vi "pH电极校准.vi"() -> ()   [LabVIEW 2016, in "斯坦道多参数.lvlib"]
uses:
  <vilib>/Utility/miscctls.llb/LVPointTypeDef.ctl
  <vilib>/Analysis/NI_AALBase.lvlib
panel:
  in  "刷新按钮":bool
  out "第三点信号值":dbl
  out "第二点信号值":dbl
  out "第一点信号值":dbl
  out "温度":dbl format="%#.2f"
  out "通讯状态":string
  out "电极状态标志":u16(ring) items=["OK", "第一点校正通过", "第二点校正通过", "校正失败,电极零点超出范围", "校正失败,电极斜率超出范围", "第三点校正通过"]
  in  "三点标液3":u16(ring)=6 caption="标液3" items=["TECH4.00", "TECH7.00", "TECH10.00", "NIST1.68", "NIST4.01", "NIST6.86", "NIST9.18", "NIST12.68"]
  in  "三点标液2":u16(ring)=5 caption="标液2" items=["TECH4.00", "TECH7.00", "TECH10.00", "NIST1.68", "NIST4.01", "NIST6.86", "NIST9.18", "NIST12.68"]
  in  "三点标液1":u16(ring)=4 caption="标液1" items=["TECH4.00", "TECH7.00", "TECH10.00", "NIST1.68", "NIST4.01", "NIST6.86", "NIST9.18", "NIST12.68"]
  out "第三点校准值":dbl
  in  "校准停止":bool
  in  "校准启动":bool
  out "第二点校准值":dbl
  out "第一点校准值":dbl
  out "提示":string
  in  "校准模式":enum16{"两点校准", "单点校准", "三点校准"}(ring)
  out "最小值":sgl format="%#.2f"
  out "最大值":sgl format="%#.2f"
  out "变异系数":dbl format="%#.6f"
  out "standard deviation":dbl caption="标准差" format="%#.2f"
  out "mean":dbl caption="均值" format="%#.2f"
  out "波形图表":sgl(graph) caption="历史曲线"
  out "当前检测值":dbl caption="测量值" format="%#.2f"
  out "标液2":dbl
  out "标液1":dbl
  out "当前信号值":dbl caption="信号值" format="%#.2f"
  out "偏移值补偿":dbl caption="pH偏移修正值" format="%#.2f"
  out "电极斜率":dbl format="%#.6f"
  out "电极零点":dbl format="%#.6f"
  # "酸碱度电极设定"
  # "℃"
  # "mV"
  # "mV"
  # "%"
  # "请选择校准模式:"
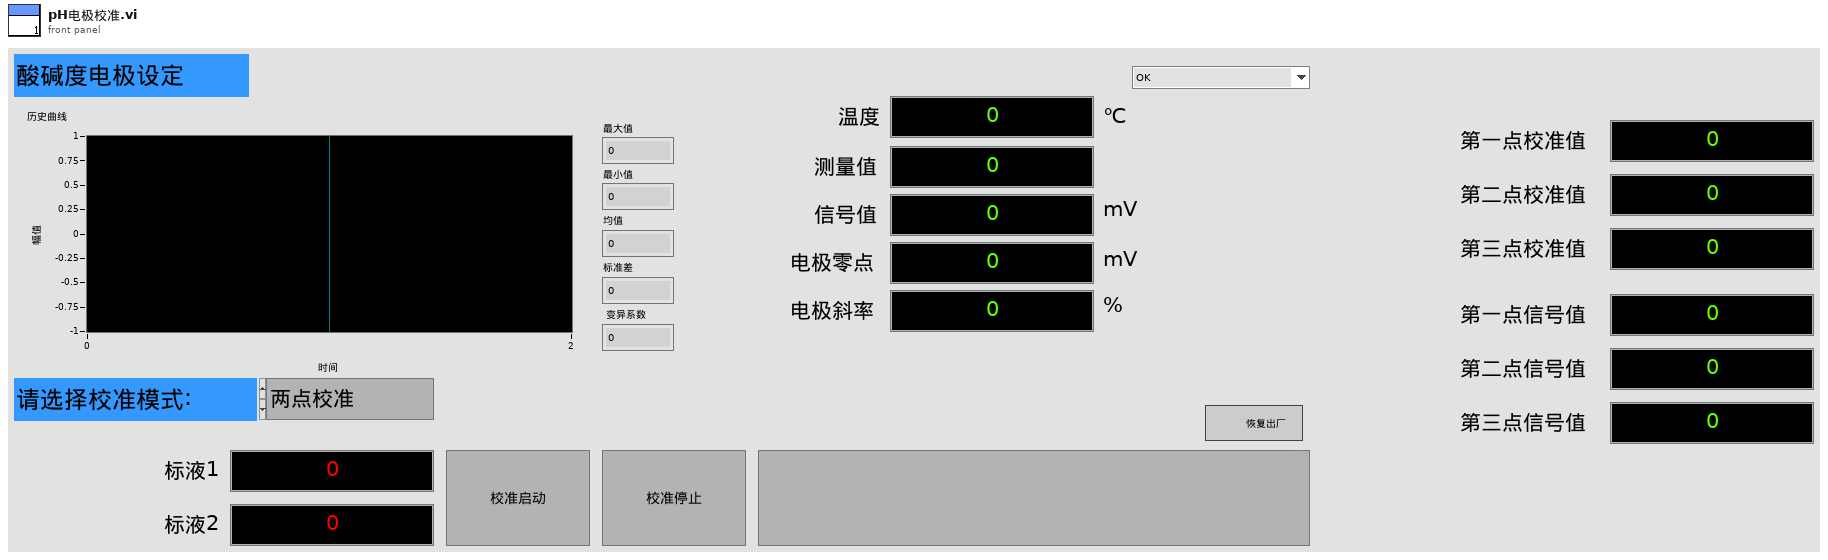
[diagram p1: front panel]
types:
  T1 = typedef "LVPointTypeDef.ctl" = cluster{"Horizontal":i16, "Vertical":i16}
  T2 = enum8{"Enabled", "Disabled", "Disabled and Grayed Out"}
  T3 = cluster{"电极状态标志":u16, "电极型号标志":u16, "酸碱度测量值":sgl, "温度测量值":sgl, "酸碱度信号值":sgl, "温度信号值":sgl, "酸碱度偏移修正值":sgl, "温度偏移修正值":sgl, "手动温度补偿值":sgl, "酸碱度电极零点":sgl, "酸碱度电极斜率":sgl, "第1点标准值记录":sgl, "第1点信号值记录":sgl, "第1点温度值记录":sgl, "第2点标准值记录":sgl, "第2点信号值记录":sgl, "第2点温度值记录":sgl, "命令滤波设定":u16, "温度模式":enum16{"ATC", "MTC"}, "生产批次":u16, "电极序号":u16, "串口地址":u16, "串口波特率":enum16{"9600", "19200", "115200"}, "串口校验位":enum16{"NONE", "ODD", "EVEN"}, "串口停止位":enum16{"1bit", "2bit"}, "第一点标准值":sgl, "第二点标准值":sgl}
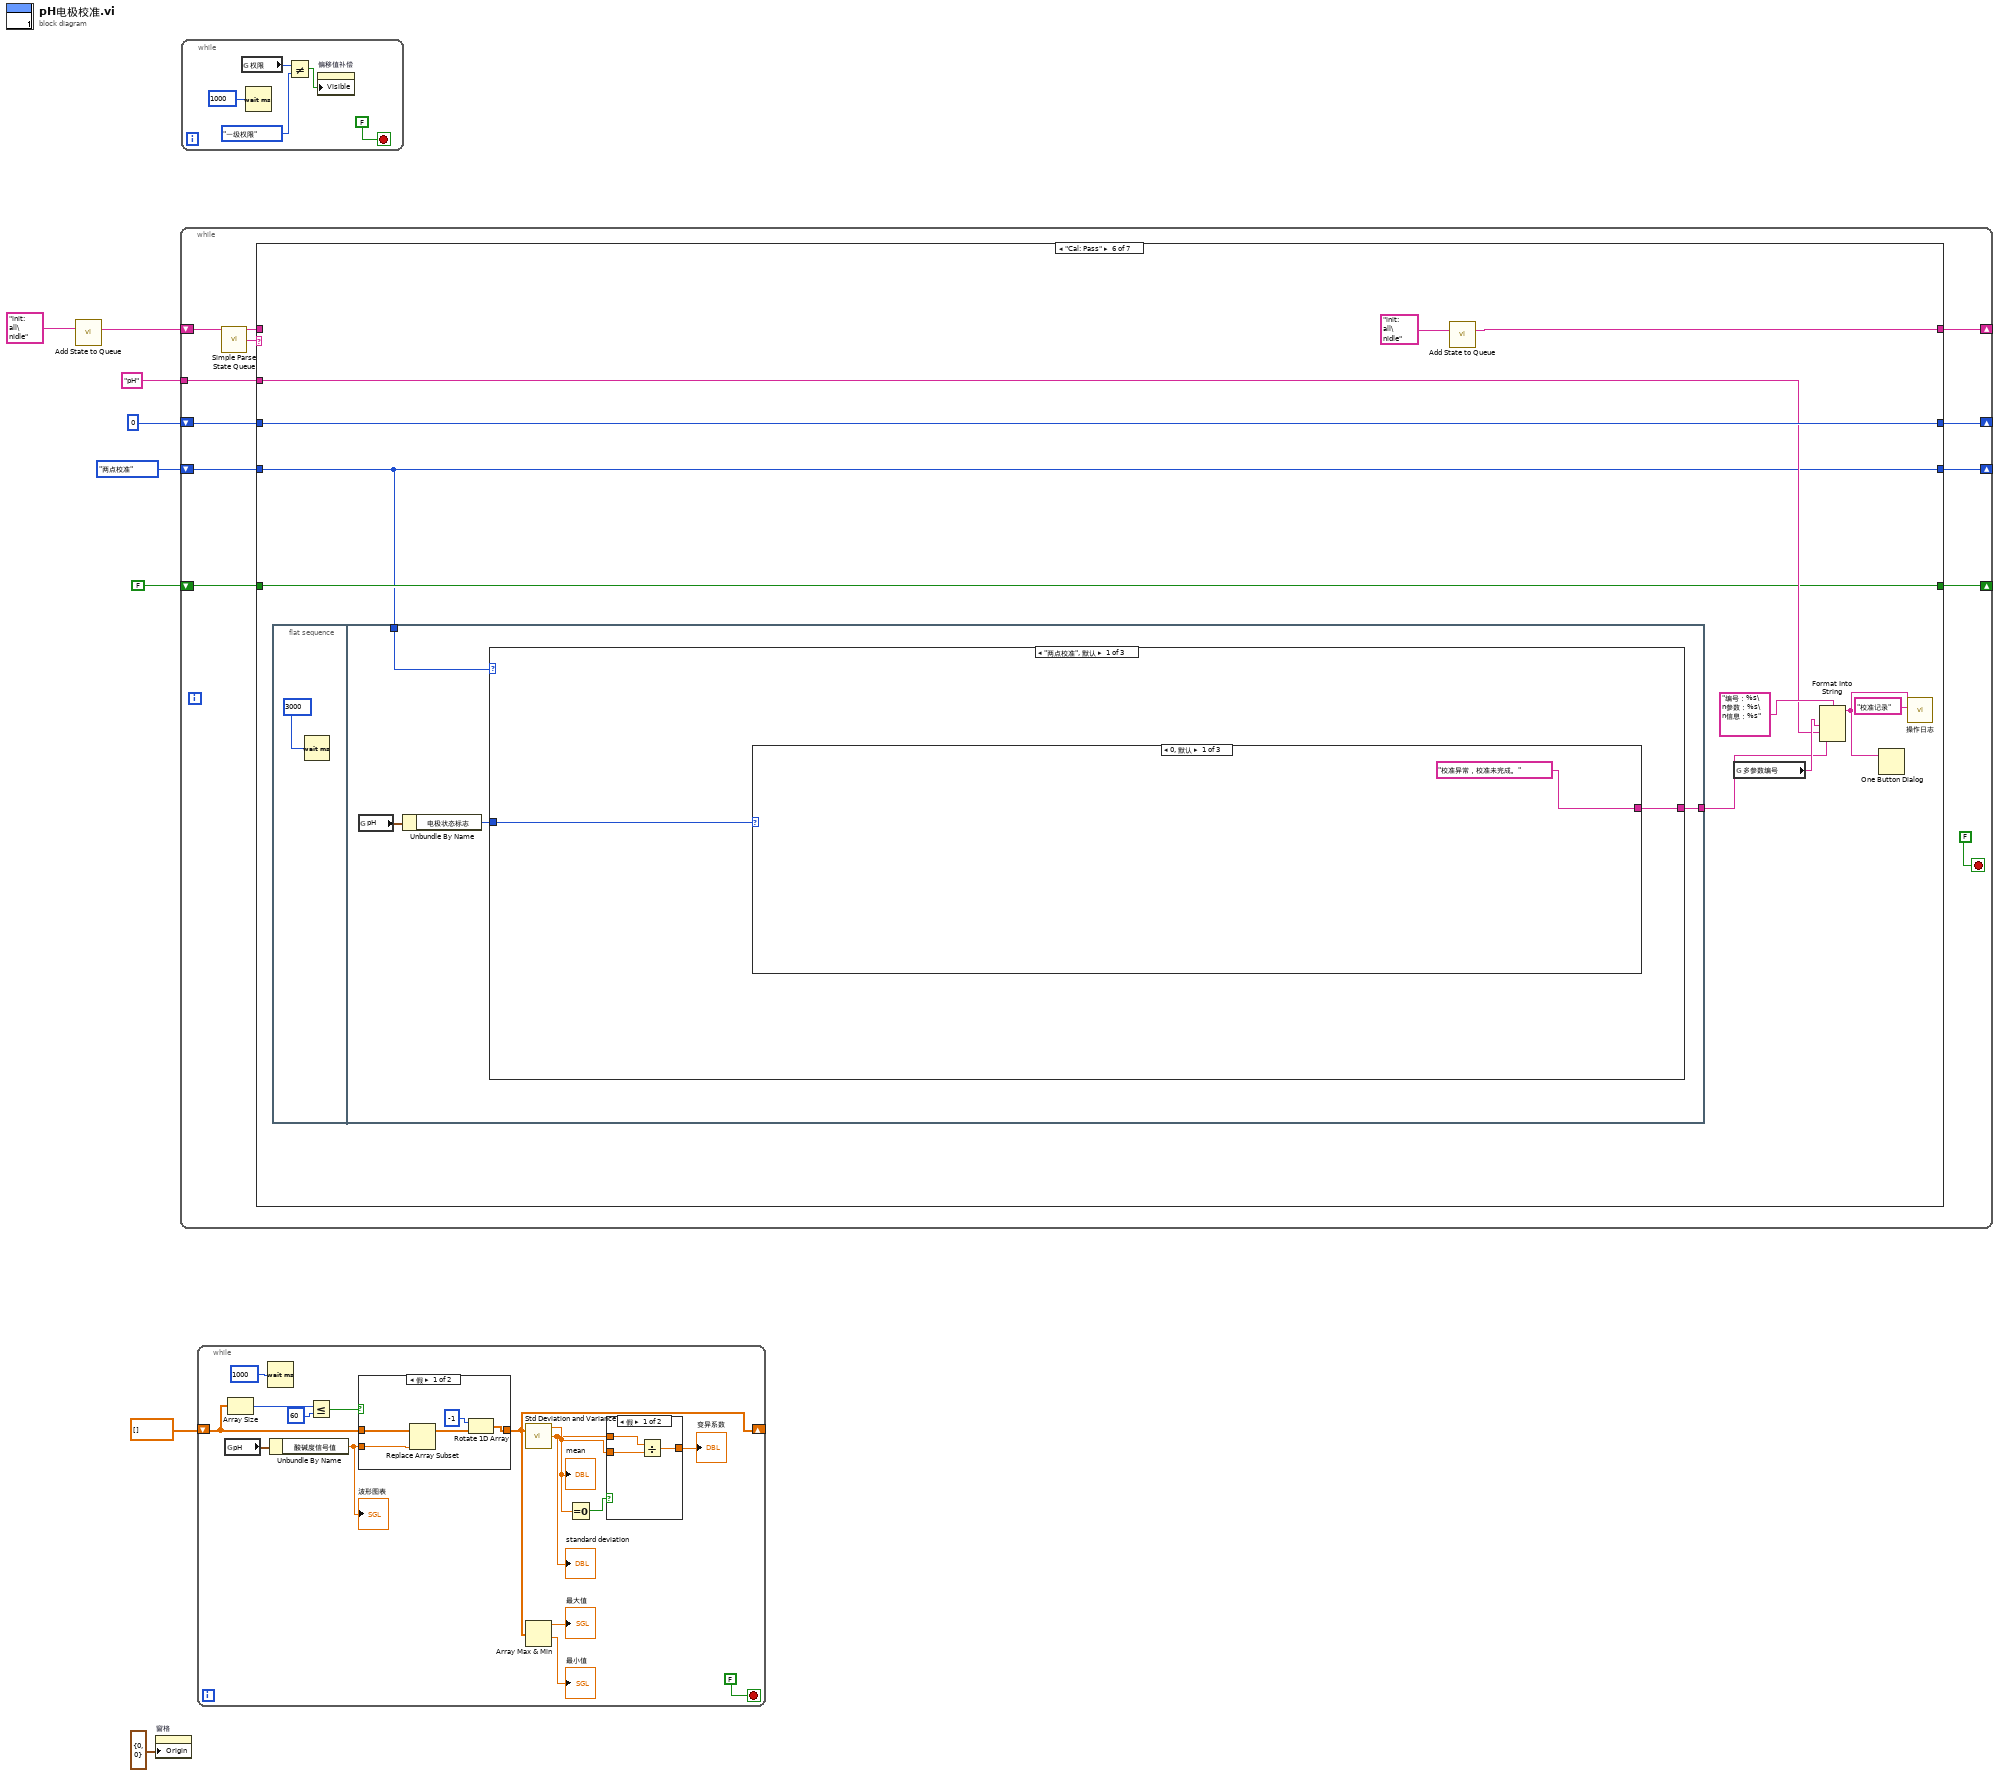
[diagram p0: block diagram]
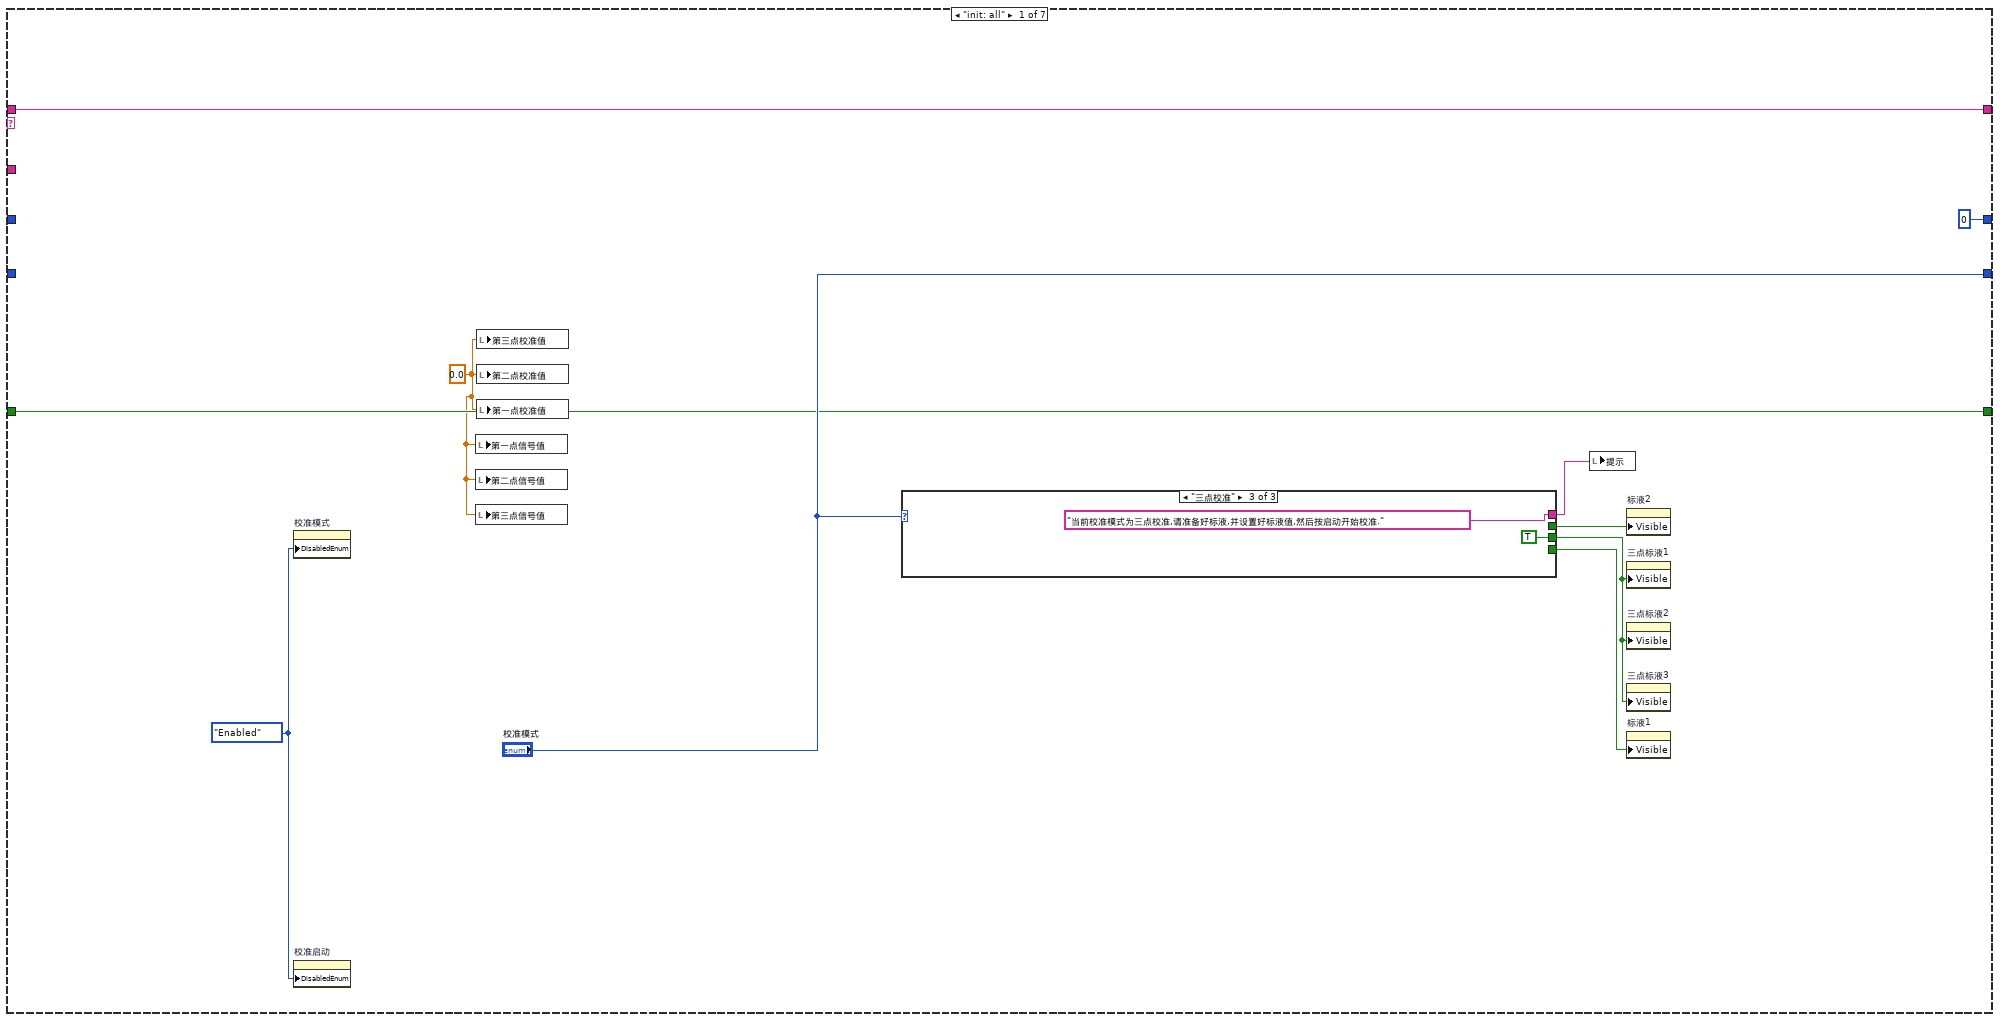
[diagram p2: hidden frame]
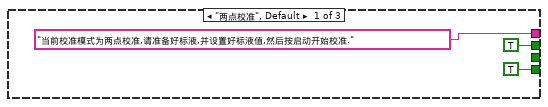
[diagram p3: hidden frame]
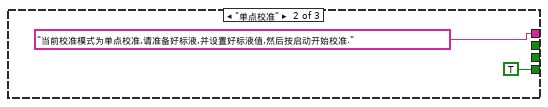
[diagram p4: hidden frame]
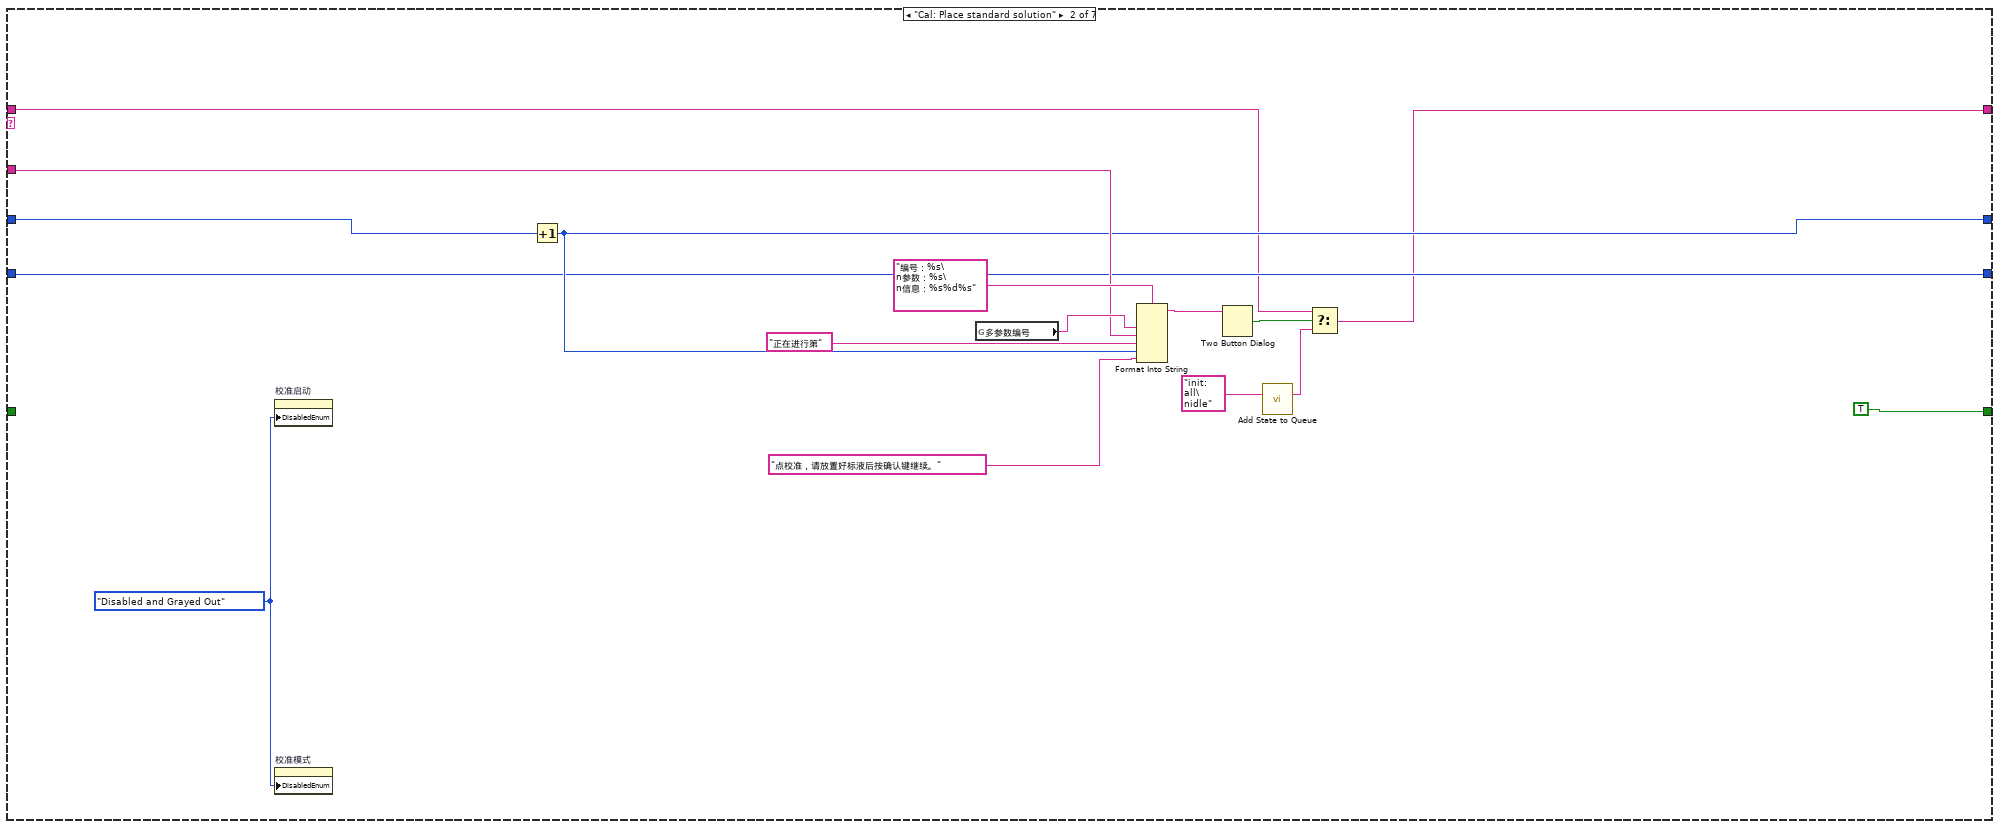
[diagram p5: hidden frame]
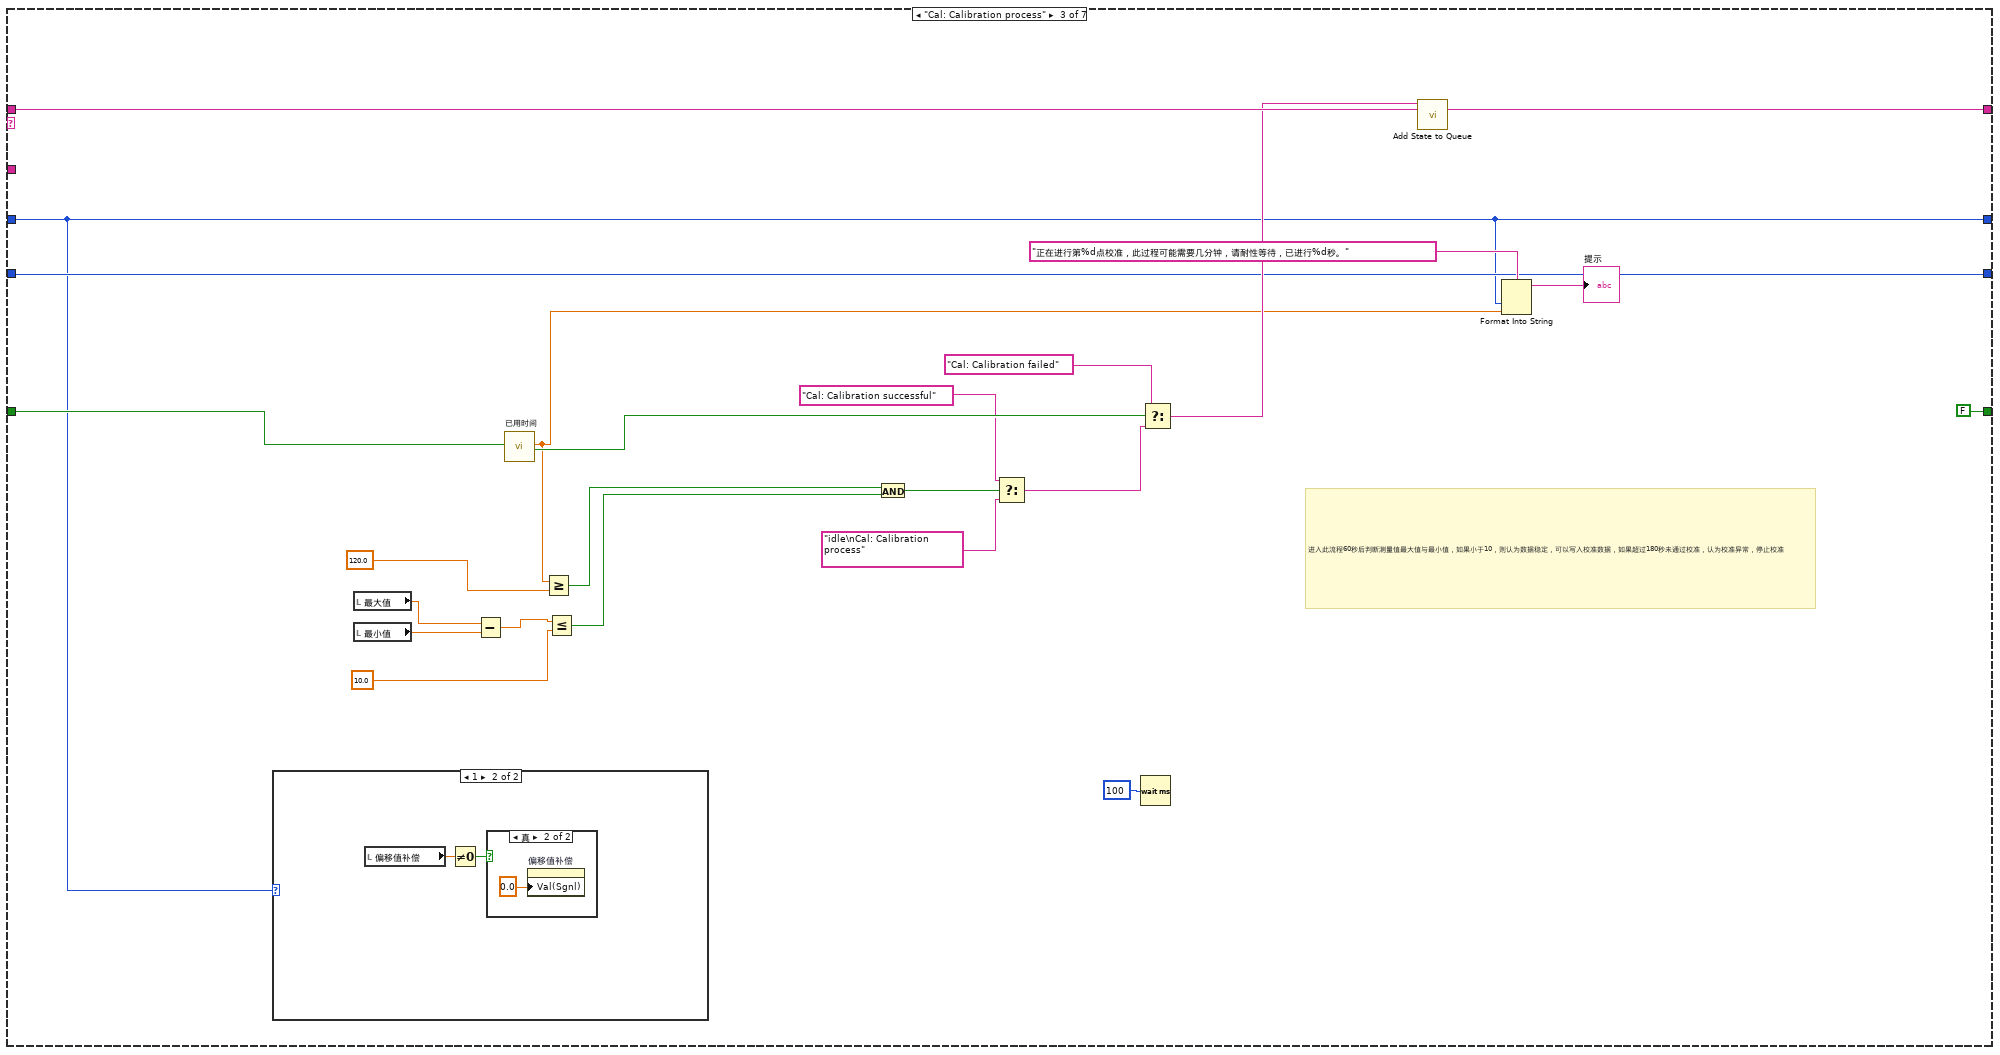
[diagram p6: hidden frame]
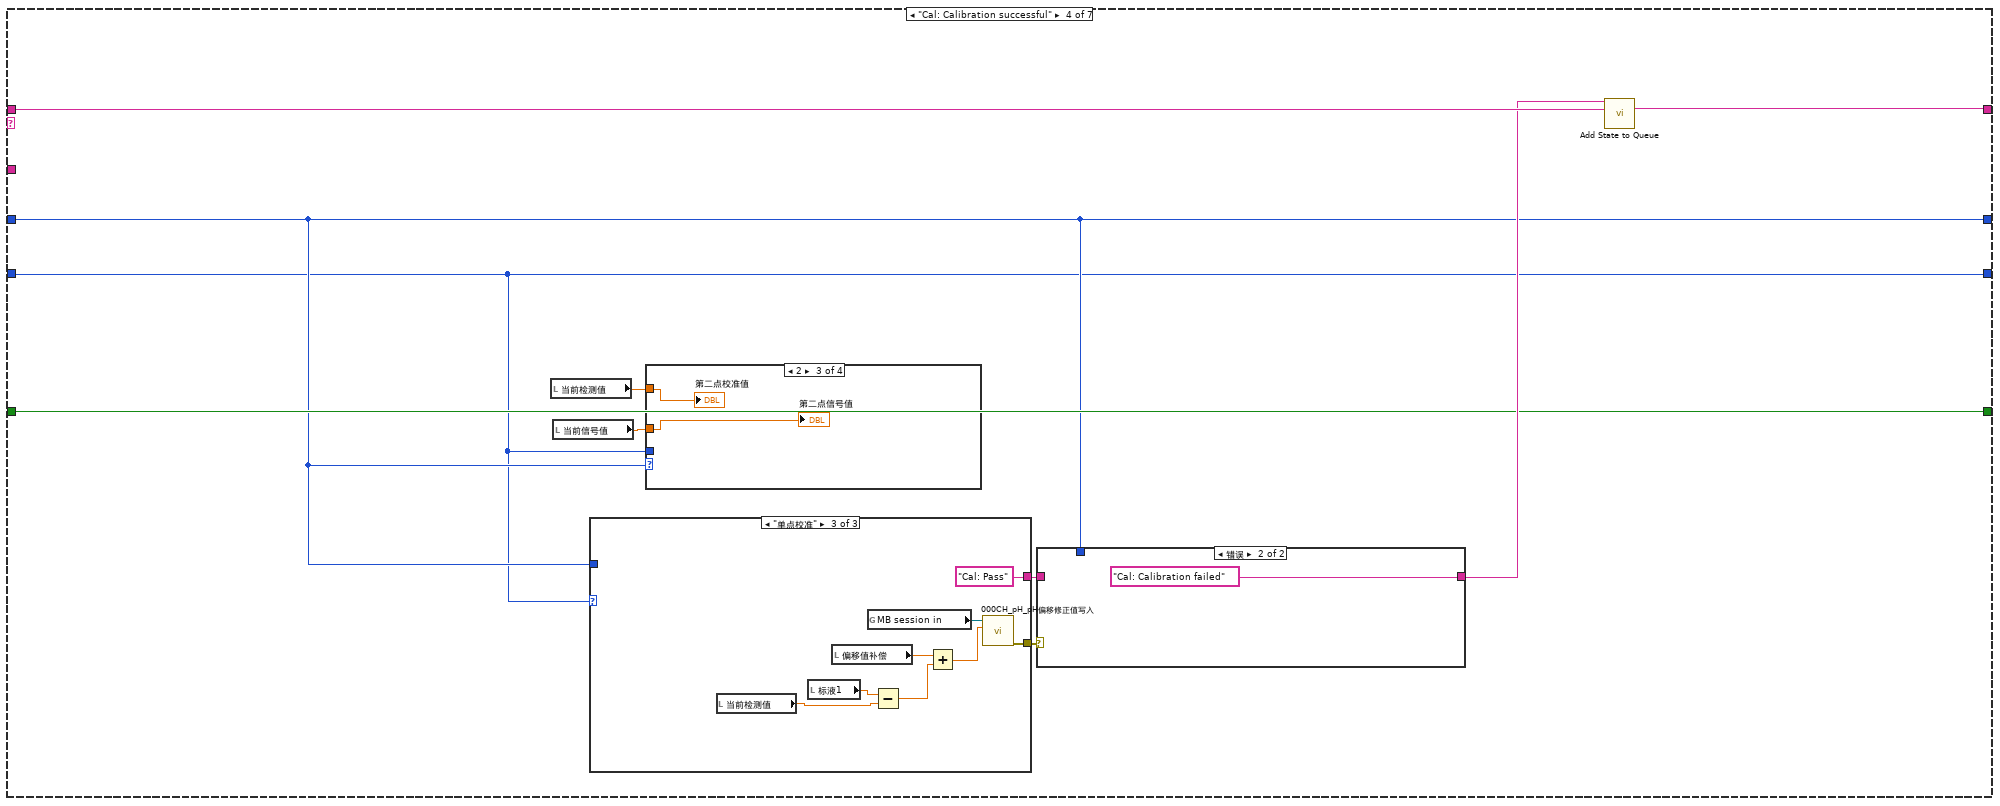
[diagram p9: hidden frame]
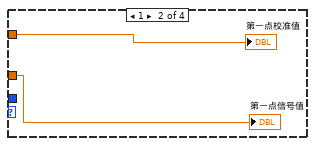
[diagram p11: hidden frame]
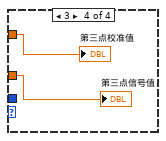
[diagram p12: hidden frame]
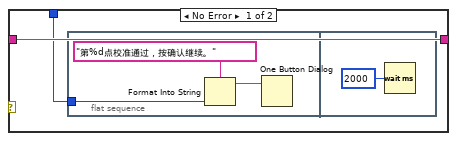
[diagram p13: hidden frame]
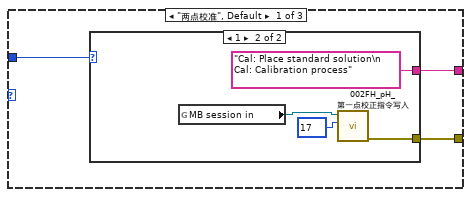
[diagram p14: hidden frame]
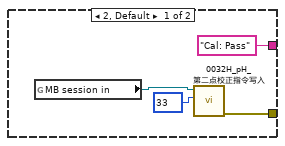
[diagram p15: hidden frame]
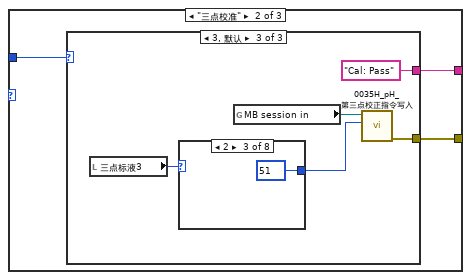
[diagram p16: hidden frame]
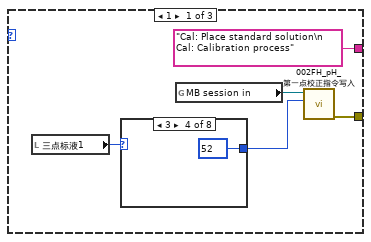
[diagram p17: hidden frame]
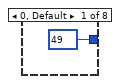
[diagram p18: hidden frame]
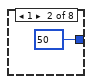
[diagram p19: hidden frame]
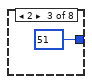
[diagram p20: hidden frame]
diagram:
  n1 = call "Add State to Queue.vi"("State(s) In (\"\")"="init: all\nidle" ("State(s) In (\"\")")) -> ("States Out"=w5:string)  [unwired: 14 in]
  n2 = property on="窗格" class="Pane"("Origin"=T1 {"Horizontal"=0, "Vertical"=0} ("原点")) -> ()  [unwired: 2 in, 2 out]
  n3 = while {
    shift-right: [w16] -> _
    shift-left: w5 -> [w20]
    shift-right: [w13] -> _
    shift-left: 0 -> [w15]
    tunnel: "pH" ("State(s) In (\"\")") -> [w14]
    shift-right: [w11] -> _
    shift-left: enum16{"两点校准", "单点校准", "三点校准"}."两点校准" ("校准模式") -> [w12]
    shift-right: [w9] -> _
    shift-left: FALSE -> [w10]
    stop <- FALSE stop-if-true
    n4 = call "Simple Parse State Queue.vi"("State Queue"=w20) -> ("Remain States"=w17:string, "Next State"=w18:string)  [unwired: 13 in]
    n5 = case shown="\"Cal: Pass\"" w18 {
      tunnel: w17 -> [w30 w39 w72 w88 _ _ w232]
      tunnel: [w30 w38 w71 w87 w172 w176 w231] -> w16
      tunnel: w15 -> [_ w49 w55 w82 w175 w186 w229]
      tunnel: w14 -> [_ w50 _ _ w165 w182 _]
      tunnel: [0 w47 w55 w82 w175 w186 w230] -> w13
      tunnel: w12 -> [_ w46 w56 w81 w174 w178 w228]
      tunnel: ["校准模式" w46 w56 w81 w174 w178 w228] -> w11
      tunnel: w10 -> [w23 _ w58 w83 w173 w181 w226]
      tunnel: [w23 TRUE FALSE w83 w173 w181 w226] -> w9
      frame "init: all" {
        w22 = T2."Enabled" ("禁用")
        w21 = 0.0 ("第一点校准值")
        n6 = property on="校准模式" class="Enum (严格)"("DisabledEnum"=w22) -> ()  [unwired: 2 in, 2 out]
        n7 = property on="校准启动" class="Bool"("DisabledEnum"=w22) -> ()  [unwired: 2 in, 2 out]
        n8 = local write "第一点信号值"(w21) -> ()
        n9 = local write "第二点信号值"(w21) -> ()
        n10 = local write "第三点信号值"(w21) -> ()
        n11 = local write "第三点校准值"(w21) -> ()
        n12 = local write "第二点校准值"(w21) -> ()
        n13 = local write "第一点校准值"(w21) -> ()
        n14 = case shown="\"三点校准\"" "校准模式" {
          tunnel: ["当前校准模式为两点校准,请准备好标液,并设置好标液值,然后按启动开始校准." ("提示") "当前校准模式为单点校准,请准备好标液,并设置好标液值,然后按启动开始校准." ("提示") "当前校准模式为三点校准,请准备好标液,并设置好标液值,然后按启动开始校准." ("提示")] -> w25
          tunnel: [TRUE ("可见") _ _] -> w29
          tunnel: [TRUE ("可见") TRUE ("可见") _] -> w27
          tunnel: [_ _ TRUE ("可见")] -> w28
          frame "两点校准", Default {
          }
          frame "单点校准" {
          }
          frame "三点校准" {
          }
        }
        n15 = local write "提示"(w25) -> ()
        n16 = property on="标液2" class="DigNum (严格)"("Visible"=w29) -> ()  [unwired: 2 in, 2 out]
        n17 = property on="三点标液1" class="Ring (严格)"("Visible"=w28) -> ()  [unwired: 2 in, 2 out]
        n18 = property on="三点标液2" class="Ring (严格)"("Visible"=w28) -> ()  [unwired: 2 in, 2 out]
        n19 = property on="三点标液3" class="Ring (严格)"("Visible"=w28) -> ()  [unwired: 2 in, 2 out]
        n20 = property on="标液1" class="DigNum (严格)"("Visible"=w27) -> ()  [unwired: 2 in, 2 out]
      }
      frame "Cal: Place standard solution" {
        w44 = T2."Disabled and Grayed Out" ("禁用")
        n21 = property on="校准启动" class="Bool"("DisabledEnum"=w44) -> ()  [unwired: 2 in, 2 out]
        n22 = property on="校准模式" class="Enum (严格)"("DisabledEnum"=w44) -> ()  [unwired: 2 in, 2 out]
        n23 = Increment(x=w49) -> (x+1=w47:i32)
        n24 = global read "多参数全局变量.vi" "多参数编号"() -> (w52:string)
        n25 = Format Into String(format string="编号：%s\n参数：%s\n信息：%s%d%s" ("格式字符串"), w52, w50, "正在进行第" ("消息"), w47, "点校准，请放置好标液后按确认键继续。" ("消息")) -> (resulting string=w43:string)  [unwired: 2 in, 1 out]
        n26 = Two Button Dialog(message=w43) -> (T button?=w42:bool)  [unwired: 2 in]
        n27 = call "Add State to Queue.vi"("State(s) In (\"\")"="init: all\nidle" ("State(s) In (\"\")")) -> ("States Out"=w40:string)  [unwired: 14 in]
        n28 = Select(t=w39, s=w42, f=w40) -> (s? t:f=w38:string)
      }
      frame "Cal: Calibration process" {
        # "进入此流程60秒后判断测量值最大值与最小值，如果小于10，则认为数据稳定，可以写入校准数据，如果超过180秒未通过校准，认为校准异常，停止校准"
        n29 = case shown="1" w55 {
          frame 0, Default {
          }
          frame 1 {
            n30 = local read "偏移值补偿"() -> (w78:dbl)
            n31 = Not Equal To 0?(x=w78) -> (x != 0?=w79:bool)
            n32 = case shown="真" w79 {
              frame False {
              }
              frame True {
                n33 = property on="偏移值补偿" class="DigNum (严格)"("Val(Sgnl)"=0.0 ("值(信号)")) -> ()  [unwired: 2 in, 2 out]
              }
            }
          }
        }
        n34 = local read "最大值"() -> (w76:sgl)
        n35 = local read "最小值"() -> (w75:sgl)
        n36 = Subtract(x=w76, y=w75) -> (x-y=w77:sgl)
        n37 = call "已用时间"("Reset"=w58) -> ("Elapsed Time (s)"=w54:dbl, "Time has Elapsed"=w73:bool)  [unwired: 11 in, 6 out]
        n38 = Greater Or Equal?(x=w54, y=120.0) -> (x >= y?=w68:bool)
        n39 = Less Or Equal?(x=w77, y=10.0) -> (x <= y?=w64:bool)
        n40 = And(x=w68, y=w64) -> (x .and. y?=w65:bool)
        n41 = Select(t="Cal: Calibration successful" ("State(s) In (\"\")"), s=w65, f="idle\nCal: Calibration process" ("State(s) In (\"\")")) -> (s? t:f=w63:string)
        n42 = Wait (ms)(milliseconds to wait=u32 100 ("等待时间（毫秒）")) -> ()  [unwired: 1 out]
        n43 = Select(t="Cal: Calibration failed" ("State(s) In (\"\")"), s=w73, f=w63) -> (s? t:f=w62:string)
        n44 = call "Add State to Queue.vi"("State(s) In Front (\"\")"=w62, "State(s) In (\"\")"=w72) -> ("States Out"=w71:string)  [unwired: 13 in]
        n45 = Format Into String(format string="正在进行第%d点校准，此过程可能需要几分钟，请耐性等待，已进行%d秒。" ("格式字符串"), w55, w54) -> (resulting string=→"提示":string)  [unwired: 2 in, 1 out]
      }
      frame "Cal: Calibration successful" {
        n46 = local read "当前检测值"() -> (w84:dbl)
        n47 = local read "当前信号值"() -> (w85:dbl)
        n48 = case shown="\"单点校准\"" w81 {
          tunnel: [w106 w117 w159] -> w90
          tunnel: [w105 w115 "Cal: Pass" ("State(s) In (\"\")")] -> w89
          tunnel: w82 -> [w104 w116 _]
          frame "两点校准", Default {
            n49 = case shown="1" w104 {
              tunnel: [w107 w112] -> w106
              tunnel: ["Cal: Pass" ("State(s) In (\"\")") "Cal: Place standard solution\n Cal: Calibration process" ("State(s) In (\"\")")] -> w105
              frame 2, Default {
                n50 = global read "多参数全局变量.vi" "MB session in"() -> (w109:refnum<class "MB_Master.lvclass">)
                n51 = call "0032H_pH_第二点校正指令写入.vi"("数值"=u16 33, "MB session in"=w109) -> ("error out"=w107:errorcluster)  [unwired: 8 in, 1 out]
              }
              frame 1 {
                n52 = global read "多参数全局变量.vi" "MB session in"() -> (w114:refnum<class "MB_Master.lvclass">)
                n53 = call "002FH_pH_第一点校正指令写入.vi"("数值"=u16 17, "MB session in"=w114) -> ("error out"=w112:errorcluster)  [unwired: 8 in, 1 out]
              }
            }
          }
          frame "三点校准" {
            n54 = case shown="3, 默认" w116 {
              tunnel: [w119 w132 w145] -> w117
              tunnel: ["Cal: Place standard solution\n Cal: Calibration process" ("State(s) In (\"\")") "Cal: Place standard solution\n Cal: Calibration process" ("State(s) In (\"\")") "Cal: Pass" ("State(s) In (\"\")")] -> w115
              frame 1 {
                n55 = local read "三点标液1"() -> (w121:u16)
                n56 = case shown="3" w121 {
                  tunnel: [u16 49 ("数值") u16 50 ("数值") u16 51 ("数值") u16 52 ("数值") u16 53 ("数值") u16 54 ("数值") u16 55 ("数值") u16 56 ("数值")] -> w120
                  frame 0, Default {
                  }
                  frame 1 {
                  }
                  frame 2 {
                  }
                  frame 3 {
                  }
                  frame 4 {
                  }
                  frame 5 {
                  }
                  frame 6 {
                  }
                  frame 7 {
                  }
                }
                n57 = global read "多参数全局变量.vi" "MB session in"() -> (w122:refnum<class "MB_Master.lvclass">)
                n58 = call "002FH_pH_第一点校正指令写入.vi"("数值"=w120, "MB session in"=w122) -> ("error out"=w119:errorcluster)  [unwired: 8 in, 1 out]
              }
              frame 2 {
                n59 = local read "三点标液2"() -> (w134:u16)
                n60 = case shown="7" w134 {
                  tunnel: [u16 49 ("数值") u16 50 ("数值") u16 51 ("数值") u16 52 ("数值") u16 53 ("数值") u16 54 ("数值") u16 55 ("数值") u16 56 ("数值")] -> w133
                  frame 0, Default {
                  }
                  frame 1 {
                  }
                  frame 2 {
                  }
                  frame 3 {
                  }
                  frame 4 {
                  }
                  frame 5 {
                  }
                  frame 6 {
                  }
                  frame 7 {
                  }
                }
                n61 = global read "多参数全局变量.vi" "MB session in"() -> (w135:refnum<class "MB_Master.lvclass">)
                n62 = call "0032H_pH_第二点校正指令写入.vi"("数值"=w133, "MB session in"=w135) -> ("error out"=w132:errorcluster)  [unwired: 8 in, 1 out]
              }
              frame 3, Default {
                n63 = local read "三点标液3"() -> (w147:u16)
                n64 = case shown="2" w147 {
                  tunnel: [u16 49 ("数值") u16 50 ("数值") u16 51 ("数值") u16 52 ("数值") u16 53 ("数值") u16 54 ("数值") u16 55 ("数值") u16 56 ("数值")] -> w146
                  frame 0, Default {
                  }
                  frame 1 {
                  }
                  frame 2 {
                  }
                  frame 3 {
                  }
                  frame 4 {
                  }
                  frame 5 {
                  }
                  frame 6 {
                  }
                  frame 7 {
                  }
                }
                n65 = global read "多参数全局变量.vi" "MB session in"() -> (w148:refnum<class "MB_Master.lvclass">)
                n66 = call "0035H_pH_第三点校正指令写入.vi"("数值"=w146, "MB session in"=w148) -> ("error out"=w145:errorcluster)  [unwired: 8 in, 1 out]
              }
            }
          }
          frame "单点校准" {
            n67 = local read "当前检测值"() -> (w157:dbl)
            n68 = local read "标液1"() -> (w164:dbl)
            n69 = local read "偏移值补偿"() -> (w160:dbl)
            n70 = global read "多参数全局变量.vi" "MB session in"() -> (w163:refnum<class "MB_Master.lvclass">)
            n71 = Subtract(x=w164, y=w157) -> (x-y=w162:dbl)
            n72 = Add(x=w160, y=w162) -> (x+y=w161:dbl)
            n73 = call "000CH_pH_pH偏移修正值写入.vi"("数值"=w161, "MB session in"=w163) -> ("error out"=w159:errorcluster)  [unwired: 8 in, 1 out]
          }
        }
        n74 = case shown="2" w82 {
          tunnel: w85 -> [_ w92 w93 w95]
          tunnel: w84 -> [_ w91 w94 w96]
          tunnel: w81 -> [_ _ _ _]
          frame 0, Default {
          }
          frame 1 {
            "第一点校准值" <- w91
            "第一点信号值" <- w92
          }
          frame 2 {
            "第二点校准值" <- w94
            "第二点信号值" <- w93
          }
          frame 3 {
            "第三点校准值" <- w96
            "第三点信号值" <- w95
          }
        }
        n75 = case shown="错误" w90 {
          tunnel: w89 -> [w98 _]
          tunnel: [w98 "Cal: Calibration failed" ("State(s) In (\"\")")] -> w86
          tunnel: w82 -> [w97 _]
          frame No Error {
            n76 = flat-sequence {
              tunnel: w97 -> [w99]
              frame #0 {
                n77 = Format Into String(format string="第%d点校准通过，按确认继续。" ("格式字符串"), w99) -> (resulting string=w101:string)  [unwired: 2 in, 1 out]
                n78 = One Button Dialog(message=w101) -> ()  [unwired: 1 in, 1 out]
              }
              frame #1 {
                n79 = Wait (ms)(milliseconds to wait=u32 2000 ("等待时间（毫秒）")) -> ()  [unwired: 1 out]
              }
            }
          }
          frame Error {
          }
        }
        n80 = call "Add State to Queue.vi"("State(s) In Front (\"\")"=w86, "State(s) In (\"\")"=w88) -> ("States Out"=w87:string)  [unwired: 13 in]
      }
      frame "Cal: Calibration failed" {
        n81 = global read "多参数全局变量.vi" "多参数编号"() -> (w168:string)
        n82 = call "Add State to Queue.vi"("State(s) In (\"\")"="init: all\nidle" ("State(s) In (\"\")")) -> ("States Out"=w172:string)  [unwired: 14 in]
        n83 = Format Into String(format string="编号：%s\n参数：%s\n信息：%s" ("格式字符串"), w168, w165, "校准失败！" ("消息")) -> (resulting string=w167:string)  [unwired: 2 in, 1 out]
        n84 = One Button Dialog(message=w167) -> ()  [unwired: 1 in, 1 out]
        n85 = call "操作日志.vi"("table"="校准记录", "日志信息"=w167) -> ()  [unwired: 9 in, 1 out]
      }
      frame "Cal: Pass" {
        n86 = flat-sequence {
          tunnel: [w189] -> w179
          tunnel: w178 -> [w188]
          frame #0 {
            n87 = Wait (ms)(milliseconds to wait=u32 3000 ("等待时间（毫秒）")) -> ()  [unwired: 1 out]
          }
          frame #1 {
            n88 = global read "国弘过程全局变量.vi" "pH"() -> (w190:T3)
            n89 = Unbundle By Name(w190) -> ("电极状态标志"=w191:u16)
            n90 = case shown="\"两点校准\", 默认" w188 {
              tunnel: [w193 w208 w225] -> w189
              tunnel: w191 -> [w192 w207 _]
              frame "两点校准", Default {
                n91 = case shown="0, 默认" w192 {
                  selector: w192 -> [_ _ w204]
                  tunnel: ["校准异常，校准未完成。" ("格式字符串") w202 w203] -> w193
                  frame 0, Default {
                  }
                  frame 2 {
                    n92 = local read "第一点校准值"() -> (w200:dbl)
                    n93 = local read "第一点信号值"() -> (w201:dbl)
                    n94 = local read "第二点校准值"() -> (w197:dbl)
                    n95 = local read "第二点信号值"() -> (w196:dbl)
                    n96 = local read "标液1"() -> (w198:dbl)
                    n97 = local read "标液2"() -> (w195:dbl)
                    n98 = Format Into String(format string="校准结果：\n第一点校准值=%#.2f，第一点信号值=%#.2f mV，第一点标准值=%#.2f；\n第二点校准值=%#.2f，第二点信号值=%#.2f mV，第二点标准值=%#.2f。" ("提示"), w200, w201, w198, w197, w196, w195) -> (resulting string=w202:string)  [unwired: 2 in, 1 out]
                  }
                  frame 3, 4 {
                    n99 = case shown="4" w204 {
                      tunnel: ["校正失败，电极零点超出范围" "校正失败，电极斜率超出范围"] -> w203
                      frame 3, Default {
                      }
                      frame 4 {
                      }
                    }
                  }
                }
              }
              frame "三点校准" {
                n100 = case shown="5" w207 {
                  tunnel: ["校准异常，校准未完成。" ("格式字符串") w220] -> w208
                  frame 0, Default {
                  }
                  frame 5 {
                    n101 = local read "第一点校准值"() -> (w219:dbl)
                    n102 = local read "第一点信号值"() -> (w217:dbl)
                    n103 = local read "第二点校准值"() -> (w215:dbl)
                    n104 = local read "第二点信号值"() -> (w214:dbl)
                    n105 = local read "第三点校准值"() -> (w212:dbl)
                    n106 = local read "第三点信号值"() -> (w211:dbl)
                    n107 = property on="三点标液1" class="Ring (严格)"() -> ("RingText.Text"=w216:string)  [unwired: 2 in, 2 out]
                    n108 = property on="三点标液2" class="Ring (严格)"() -> ("RingText.Text"=w213:string)  [unwired: 2 in, 2 out]
                    n109 = property on="三点标液3" class="Ring (严格)"() -> ("RingText.Text"=w210:string)  [unwired: 2 in, 2 out]
                    n110 = Format Into String(format string="校准结果：\n第一点校准值=%#.2f，第一点信号值=%#.2f mV，第一点标准值=%s；\n第二点校准值=%#.2f，第二点信号值=%#.2f mV，第二点标准值=%s；\n第三点校准值=%#.2f，第三点信号值=%#.2f mV，第三点标准值=%s。" ("提示"), w219, w217, w216, w215, w214, w213, w212, w211, w210) -> (resulting string=w220:string)  [unwired: 2 in, 1 out]
                  }
                }
              }
              frame "单点校准" {
                n111 = local read "第一点校准值"() -> (w224:dbl)
                n112 = local read "第一点信号值"() -> (w222:dbl)
                n113 = local read "标液1"() -> (w221:dbl)
                n114 = Format Into String(format string="校准结果：\n校准值=%#.2f，信号值=%#.2f，标准值=%#.2f。" ("提示"), w224, w222, w221) -> (resulting string=w225:string)  [unwired: 2 in, 1 out]
              }
            }
          }
        }
        n115 = call "Add State to Queue.vi"("State(s) In (\"\")"="init: all\nidle" ("State(s) In (\"\")")) -> ("States Out"=w176:string)  [unwired: 14 in]
        n116 = global read "多参数全局变量.vi" "多参数编号"() -> (w183:string)
        n117 = Format Into String(format string="编号：%s\n参数：%s\n信息：%s" ("格式字符串"), w183, w182, w179) -> (resulting string=w180:string)  [unwired: 2 in, 1 out]
        n118 = One Button Dialog(message=w180) -> ()  [unwired: 1 in, 1 out]
        n119 = call "操作日志.vi"("table"="校准记录", "日志信息"=w180) -> ()  [unwired: 9 in, 1 out]
      }
      frame "idle", Default {
        n120 = event shown="[10] \"校准启动\": 值改变" {
          selector: _ -> [_ _ _ _ _ _ _ _ _ _ _ _]
          dyn-events: _ -> [_ _ _ _ _ _ _ _ _ _ _ _]
          timeout: 10 -> [_ _ _ _ _ _ _ _ _ _ _ _]
          tunnel: [_ _ _ _ _ _ w317 w327 w333 _ _ _] -> _
          tunnel: w232 -> [w249 w253 w254 w276 w290 w308 w322 w323 w329 w337 w345 _]
          tunnel: [w248 w252 w255 w277 w291 w309 w321 w324 w330 w336 w344 w347] -> w231
          tunnel: [w247 w250 w256 w278 w292 w311 w320 w325 w331 w335 w342 w348] -> w230
          tunnel: w229 -> [w247 w250 w256 w278 w292 w311 w320 w325 w331 w335 w342 w348]
          event Timeout {
            n121 = event-data() -> ()  [unwired: 1 in, 3 out]
            n122 = global read "国弘过程全局变量.vi" "pH"() -> (w246:T3)
            n123 = Unbundle By Name(w246) -> ("电极状态标志"=→"电极状态标志":u16, "酸碱度电极零点"=→"电极零点":sgl, "酸碱度电极斜率"=→"电极斜率":sgl, "酸碱度偏移修正值"=→"偏移值补偿":sgl, "酸碱度信号值"=→"当前信号值":sgl, "第一点标准值"=→"标液1":sgl, "第二点标准值"=→"标液2":sgl, "酸碱度测量值"=→"当前检测值":sgl, "温度测量值"=→"温度":sgl)  [unwired: 1 out]
            n124 = global read "多参数全局变量.vi" "ph通讯状态"() -> (w235:bool)
            n125 = property on="通讯状态" class="Str"("Blinking"=TRUE ("闪烁"), "Text.BG Color"=u32 16711680, "Visible"=w235) -> ()  [unwired: 2 in, 2 out]
            n126 = call "Add State to Queue.vi"("State(s) In (\"\")"=w249) -> ("States Out"=w248:string)  [unwired: 14 in]
            "通讯状态" <- "通讯异常" ("当前串口")
          }
          event "校准模式": Value Change {
            n127 = event-data() -> ()  [unwired: 1 in, 6 out]
            n128 = call "Add State to Queue.vi"("State(s) In (\"\")"=w253, "State(s) At Back (\"\")"="init: all\nidle" ("State(s) In (\"\")")) -> ("States Out"=w252:string)  [unwired: 13 in]
          }
          event "三点标液1": Value Change {
            n129 = event-data() -> ("NewVal"=w257:u16)  [unwired: 1 in, 5 out]
            n130 = case shown="1" w257 {
              frame 0, Default {
                w258 = u16 0 items=["TECH4.00", "TECH7.00", "TECH10.00", "NIST1.68", "NIST4.01", "NIST6.86", "NIST9.18", "NIST12.68"] ("标液2")
                w259 = u16 2 items=["TECH4.00", "TECH7.00", "TECH10.00", "NIST1.68", "NIST4.01", "NIST6.86", "NIST9.18", "NIST12.68"] ("标液3")
                w260 = u16 1 items=["TECH4.00", "TECH7.00", "TECH10.00", "NIST1.68", "NIST4.01", "NIST6.86", "NIST9.18", "NIST12.68"] ("标液2")
                n131 = local write "三点标液3"(w259) -> ()
                n132 = local write "三点标液2"(w260) -> ()
                n133 = local write "三点标液1"(w258) -> ()
              }
              frame 1 {
                w261 = u16 0 items=["TECH4.00", "TECH7.00", "TECH10.00", "NIST1.68", "NIST4.01", "NIST6.86", "NIST9.18", "NIST12.68"] ("标液2")
                w262 = u16 2 items=["TECH4.00", "TECH7.00", "TECH10.00", "NIST1.68", "NIST4.01", "NIST6.86", "NIST9.18", "NIST12.68"] ("标液3")
                w263 = u16 1 items=["TECH4.00", "TECH7.00", "TECH10.00", "NIST1.68", "NIST4.01", "NIST6.86", "NIST9.18", "NIST12.68"] ("标液2")
                n134 = local write "三点标液3"(w262) -> ()
                n135 = local write "三点标液2"(w263) -> ()
                n136 = local write "三点标液1"(w261) -> ()
              }
              frame 2 {
                w264 = u16 2 items=["TECH4.00", "TECH7.00", "TECH10.00", "NIST1.68", "NIST4.01", "NIST6.86", "NIST9.18", "NIST12.68"] ("标液2")
                w265 = u16 0 items=["TECH4.00", "TECH7.00", "TECH10.00", "NIST1.68", "NIST4.01", "NIST6.86", "NIST9.18", "NIST12.68"] ("标液3")
                w266 = u16 1 items=["TECH4.00", "TECH7.00", "TECH10.00", "NIST1.68", "NIST4.01", "NIST6.86", "NIST9.18", "NIST12.68"] ("标液2")
                n137 = local write "三点标液3"(w265) -> ()
                n138 = local write "三点标液2"(w266) -> ()
                n139 = local write "三点标液1"(w264) -> ()
              }
              frame 3 {
                w267 = u16 3 items=["TECH4.00", "TECH7.00", "TECH10.00", "NIST1.68", "NIST4.01", "NIST6.86", "NIST9.18", "NIST12.68"] ("标液2")
                w268 = u16 5 items=["TECH4.00", "TECH7.00", "TECH10.00", "NIST1.68", "NIST4.01", "NIST6.86", "NIST9.18", "NIST12.68"] ("标液3")
                w269 = u16 4 items=["TECH4.00", "TECH7.00", "TECH10.00", "NIST1.68", "NIST4.01", "NIST6.86", "NIST9.18", "NIST12.68"] ("标液2")
                n140 = local write "三点标液3"(w268) -> ()
                n141 = local write "三点标液2"(w269) -> ()
                n142 = local write "三点标液1"(w267) -> ()
              }
              frame 4 {
                w270 = u16 4 items=["TECH4.00", "TECH7.00", "TECH10.00", "NIST1.68", "NIST4.01", "NIST6.86", "NIST9.18", "NIST12.68"] ("标液2")
                w271 = u16 6 items=["TECH4.00", "TECH7.00", "TECH10.00", "NIST1.68", "NIST4.01", "NIST6.86", "NIST9.18", "NIST12.68"] ("标液3")
                w272 = u16 5 items=["TECH4.00", "TECH7.00", "TECH10.00", "NIST1.68", "NIST4.01", "NIST6.86", "NIST9.18", "NIST12.68"] ("标液2")
                n143 = local write "三点标液3"(w271) -> ()
                n144 = local write "三点标液2"(w272) -> ()
                n145 = local write "三点标液1"(w270) -> ()
              }
              frame 5..7 {
                w273 = u16 5 items=["TECH4.00", "TECH7.00", "TECH10.00", "NIST1.68", "NIST4.01", "NIST6.86", "NIST9.18", "NIST12.68"] ("标液2")
                w274 = u16 7 items=["TECH4.00", "TECH7.00", "TECH10.00", "NIST1.68", "NIST4.01", "NIST6.86", "NIST9.18", "NIST12.68"] ("标液3")
                w275 = u16 6 items=["TECH4.00", "TECH7.00", "TECH10.00", "NIST1.68", "NIST4.01", "NIST6.86", "NIST9.18", "NIST12.68"] ("标液2")
                n146 = local write "三点标液3"(w274) -> ()
                n147 = local write "三点标液2"(w275) -> ()
                n148 = local write "三点标液1"(w273) -> ()
              }
            }
            n149 = call "Add State to Queue.vi"("State(s) In (\"\")"=w254) -> ("States Out"=w255:string)  [unwired: 14 in]
          }
          event "三点标液2": Value Change {
            n150 = event-data() -> ("NewVal"=w279:u16)  [unwired: 1 in, 5 out]
            n151 = case shown="6, 7" w279 {
              frame 0..2, Default {
                w280 = u16 0 items=["TECH4.00", "TECH7.00", "TECH10.00", "NIST1.68", "NIST4.01", "NIST6.86", "NIST9.18", "NIST12.68"] ("标液2")
                w281 = u16 2 items=["TECH4.00", "TECH7.00", "TECH10.00", "NIST1.68", "NIST4.01", "NIST6.86", "NIST9.18", "NIST12.68"] ("标液3")
                w282 = u16 1 items=["TECH4.00", "TECH7.00", "TECH10.00", "NIST1.68", "NIST4.01", "NIST6.86", "NIST9.18", "NIST12.68"] ("标液2")
                n152 = local write "三点标液3"(w281) -> ()
                n153 = local write "三点标液2"(w282) -> ()
                n154 = local write "三点标液1"(w280) -> ()
              }
              frame 3, 4 {
                w283 = u16 3 items=["TECH4.00", "TECH7.00", "TECH10.00", "NIST1.68", "NIST4.01", "NIST6.86", "NIST9.18", "NIST12.68"] ("标液2")
                w284 = u16 5 items=["TECH4.00", "TECH7.00", "TECH10.00", "NIST1.68", "NIST4.01", "NIST6.86", "NIST9.18", "NIST12.68"] ("标液3")
                w285 = u16 4 items=["TECH4.00", "TECH7.00", "TECH10.00", "NIST1.68", "NIST4.01", "NIST6.86", "NIST9.18", "NIST12.68"] ("标液2")
                n155 = local write "三点标液3"(w284) -> ()
                n156 = local write "三点标液2"(w285) -> ()
                n157 = local write "三点标液1"(w283) -> ()
              }
              frame 5 {
                w286 = u16 6 items=["TECH4.00", "TECH7.00", "TECH10.00", "NIST1.68", "NIST4.01", "NIST6.86", "NIST9.18", "NIST12.68"] ("标液3")
                w287 = u16 5 items=["TECH4.00", "TECH7.00", "TECH10.00", "NIST1.68", "NIST4.01", "NIST6.86", "NIST9.18", "NIST12.68"] ("标液2")
                n158 = local write "三点标液3"(w286) -> ()
                n159 = local write "三点标液2"(w287) -> ()
              }
              frame 6, 7 {
                w288 = u16 7 items=["TECH4.00", "TECH7.00", "TECH10.00", "NIST1.68", "NIST4.01", "NIST6.86", "NIST9.18", "NIST12.68"] ("标液3")
                w289 = u16 6 items=["TECH4.00", "TECH7.00", "TECH10.00", "NIST1.68", "NIST4.01", "NIST6.86", "NIST9.18", "NIST12.68"] ("标液2")
                n160 = local write "三点标液3"(w288) -> ()
                n161 = local write "三点标液2"(w289) -> ()
              }
            }
            n162 = call "Add State to Queue.vi"("State(s) In (\"\")"=w276) -> ("States Out"=w277:string)  [unwired: 14 in]
          }
          event "三点标液3": Value Change {
            n163 = event-data() -> ("NewVal"=w293:u16)  [unwired: 1 in, 5 out]
            n164 = case shown="3..7" w293 {
              frame 0, 1, Default {
                w294 = u16 2 items=["TECH4.00", "TECH7.00", "TECH10.00", "NIST1.68", "NIST4.01", "NIST6.86", "NIST9.18", "NIST12.68"] ("标液2")
                w295 = u16 0 items=["TECH4.00", "TECH7.00", "TECH10.00", "NIST1.68", "NIST4.01", "NIST6.86", "NIST9.18", "NIST12.68"] ("标液3")
                w296 = u16 1 items=["TECH4.00", "TECH7.00", "TECH10.00", "NIST1.68", "NIST4.01", "NIST6.86", "NIST9.18", "NIST12.68"] ("标液2")
                n165 = local write "三点标液3"(w295) -> ()
                n166 = local write "三点标液2"(w296) -> ()
                n167 = local write "三点标液1"(w294) -> ()
              }
              frame 2 {
                w297 = u16 0 items=["TECH4.00", "TECH7.00", "TECH10.00", "NIST1.68", "NIST4.01", "NIST6.86", "NIST9.18", "NIST12.68"] ("标液2")
                w298 = u16 2 items=["TECH4.00", "TECH7.00", "TECH10.00", "NIST1.68", "NIST4.01", "NIST6.86", "NIST9.18", "NIST12.68"] ("标液3")
                w299 = u16 1 items=["TECH4.00", "TECH7.00", "TECH10.00", "NIST1.68", "NIST4.01", "NIST6.86", "NIST9.18", "NIST12.68"] ("标液2")
                n168 = local write "三点标液3"(w298) -> ()
                n169 = local write "三点标液2"(w299) -> ()
                n170 = local write "三点标液1"(w297) -> ()
              }
              frame 3..7 {
                n171 = local read "三点标液1"() -> (w302:u16)
                n172 = local read "三点标液2"() -> (w301:u16)
                n173 = Less?(x=w302, y=w301) -> (x < y?=w300:bool)
                n174 = case shown="假" w300 {
                  frame False {
                  }
                  frame True {
                    n175 = local read "三点标液3"() -> (w305:u16)
                    n176 = local read "三点标液2"() -> (w303:u16)
                    n177 = Less Or Equal?(x=w305, y=w303) -> (x <= y?=w304:bool)
                    n178 = case shown="真" w304 {
                      tunnel: w303 -> [_ w307]
                      frame False {
                      }
                      frame True {
                        n179 = Increment(x=w307) -> (x+1=w306:u16)
                        n180 = local write "三点标液3"(w306) -> ()
                      }
                    }
                  }
                }
              }
            }
            n181 = call "Add State to Queue.vi"("State(s) In (\"\")"=w290) -> ("States Out"=w291:string)  [unwired: 14 in]
          }
          event "标液1", "标液2", "偏移值补偿": Mouse Down {
            n182 = event-data() -> ("CtlRef"=w312:refnum<vi>)  [unwired: 1 in, 7 out]
            n183 = property on="校准模式" class="Enum (严格)"() -> ("DisabledEnum"=w310:T2)  [unwired: 2 in, 2 out]
            n184 = case shown="\"Enabled\"" w310 {
              tunnel: w312 -> [w316 _]
              frame "Enabled" {
                n185 = property class="DigNum (严格)"(reference=w316) -> (reference out=w313:refnum<vi>, "Value"=w314:dbl)  [unwired: 1 in, 1 out]
                n186 = call "数字键盘.vi"("OldNumber"=w314) -> ("NewNumber"=w315:dbl)  [unwired: 1 in]
                n187 = property class="DigNum (严格)"(reference=w313, "Val(Sgnl)"=w315) -> ()  [unwired: 1 in, 2 out]
              }
              frame "Disabled", Default {
              }
            }
            n188 = call "Add State to Queue.vi"("State(s) In (\"\")"=w308) -> ("States Out"=w309:string)  [unwired: 14 in]
          }
          event "偏移值补偿": Value Change {
            n189 = event-data() -> ("NewVal"=w318:dbl)  [unwired: 1 in, 5 out]
            n190 = global read "多参数全局变量.vi" "MB session in"() -> (w319:refnum<class "MB_Master.lvclass">)
            n191 = call "000CH_pH_pH偏移修正值写入.vi"("数值"=w318, "MB session in"=w319) -> ("error out"=w317:errorcluster)  [unwired: 8 in, 1 out]
            n192 = call "Add State to Queue.vi"("State(s) In (\"\")"=w322) -> ("States Out"=w321:string)  [unwired: 14 in]
          }
          event "标液1": Value Change {
            n193 = event-data() -> ("NewVal"=w328:dbl)  [unwired: 1 in, 5 out]
            n194 = global read "多参数全局变量.vi" "MB session in"() -> (w326:refnum<class "MB_Master.lvclass">)
            n195 = call "0030H_pH_第一点标准值写入.vi"("数值"=w328, "MB session in"=w326) -> ("error out"=w327:errorcluster)  [unwired: 8 in, 1 out]
            n196 = call "Add State to Queue.vi"("State(s) In (\"\")"=w323) -> ("States Out"=w324:string)  [unwired: 14 in]
          }
          event "标液2": Value Change {
            n197 = event-data() -> ("NewVal"=w334:dbl)  [unwired: 1 in, 5 out]
            n198 = global read "多参数全局变量.vi" "MB session in"() -> (w332:refnum<class "MB_Master.lvclass">)
            n199 = call "Add State to Queue.vi"("State(s) In (\"\")"=w329) -> ("States Out"=w330:string)  [unwired: 14 in]
            n200 = call "0033H_pH_第二点标准值写入.vi"("数值"=w334, "MB session in"=w332) -> ("error out"=w333:errorcluster)  [unwired: 8 in, 1 out]
          }
          event "刷新按钮": Value Change {
            n201 = event-data() -> ()  [unwired: 1 in, 6 out]
            n202 = call "Add State to Queue.vi"("State(s) In (\"\")"=w337) -> ("States Out"=w336:string)  [unwired: 14 in]
            n203 = Two Button Dialog(message="请再次确实是否恢复出厂设置！" ("消息")) -> (T button?=w339:bool)  [unwired: 2 in]
            n204 = case shown="真" w339 {
              frame False {
              }
              frame True {
                w340 = u16 33 items=["Factory Reset"=33] ("数值")
                n205 = global read "多参数全局变量.vi" "MB session in"() -> (w341:refnum<class "MB_Master.lvclass">)
                n206 = call "0026H_pH_命令寄存器写入.vi"("数值"=w340, "MB session in"=w341) -> ()  [unwired: 8 in, 2 out]
              }
            }
          }
          event "校准启动": Value Change {
            n207 = event-data() -> ()  [unwired: 1 in, 6 out]
            n208 = call "Add State to Queue.vi"("State(s) In (\"\")"=w345, "State(s) At Back (\"\")"="init: all\nCal: Place standard solution\n Cal: Calibration process\nidle" ("State(s) In (\"\")")) -> ("States Out"=w344:string)  [unwired: 13 in]
          }
          event "校准停止": Value Change {
            n209 = event-data() -> ()  [unwired: 1 in, 6 out]
            n210 = call "Add State to Queue.vi"("State(s) In (\"\")"="init: all\nidle" ("State(s) In (\"\")")) -> ("States Out"=w347:string)  [unwired: 14 in]
          }
        }
      }
    }
  }
  n211 = while {
    stop <- FALSE stop-if-true
    n212 = global read "多参数全局变量.vi" "权限"() -> (w352:enum16{"一级权限", "二级权限", "三级权限"})
    n213 = Wait (ms)(milliseconds to wait=u32 1000 ("等待时间（毫秒）")) -> ()  [unwired: 1 out]
    n214 = Not Equal?(x=w352, y=enum16{"一级权限", "二级权限", "三级权限"}."一级权限") -> (x != y?=w350:bool)
    n215 = property on="偏移值补偿" class="DigNum (严格)"("Visible"=w350) -> ()  [unwired: 2 in, 2 out]
  }
  n216 = while {
    shift-right: [w360] -> _
    shift-left: sgl[] [] -> [w364]
    stop <- FALSE stop-if-true
    n217 = global read "国弘过程全局变量.vi" "pH"() -> (w361:T3)
    n218 = Array Size(array=w364) -> (size(s)=w366:i32)
    n219 = Wait (ms)(milliseconds to wait=u32 1000 ("等待时间（毫秒）")) -> ()  [unwired: 1 out]
    n220 = Unbundle By Name(w361) -> ("酸碱度信号值"=w354:sgl)
    "波形图表" <- w354
    n221 = Less Or Equal?(x=w366, y=60) -> (x <= y?=w365:bool)
    n222 = case shown="假" w365 {
      tunnel: w364 -> [w376 w379]
      tunnel: w354 -> [w374 w378]
      tunnel: [w372 w377] -> w360
      frame False {
        n223 = Replace Array Subset(array=w376, new element=w374) -> (w375:sgl[])  [unwired: 1 in]
        n224 = Rotate 1D Array(1:w375, 2:-1 ("n")) -> (0:w372:sgl[])
      }
      frame True {
        n225 = Insert Into Array(array=w379, new element=w378) -> (w377:sgl[])  [unwired: 1 in]
      }
    }
    n226 = call <vilib>:"Std Deviation and Variance.vi"("X"=w360) -> ("mean"=w356:dbl, "standard deviation"=w355:dbl)  [unwired: 1 in, 1 out]
    "mean" <- w356
    "standard deviation" <- w355
    n227 = Array Max & Min(array=w360) -> (max value=→"最大值":sgl, min value=→"最小值":sgl)  [unwired: 2 out]
    n228 = Equal To 0?(x=w356) -> (x = 0?=w363:bool)
    n229 = case shown="假" w363 {
      tunnel: w355 -> [w371 _]
      tunnel: [w370 _] -> w357
      tunnel: w356 -> [w369 _]
      frame False {
        n230 = Divide(x=w371, y=w369) -> (x/y=w370:dbl)
      }
      frame True {
      }
    }
    "变异系数" <- w357
  }
